vi "createTSR.vi"(0 "reference in":refnum<class "Project Panels.lvclass">=refnum, 5 "data":string[][](array[string]), 11 "error in (no error)":errorcluster) -> (4 "reference out":refnum<class "Project Panels.lvclass">, 8 "saved?":bool=TRUE, 15 "error out":errorcluster)   [LabVIEW 2015, in "Project Panels.lvclass"]
uses:
  Project Panels.lvclass
  tsrState.ctl
  SYS/File Controller_llb/File Controller.lvclass
  APP/excelFile_class/excelFile.lvclass
panel:
  out "PDF_path":path
  out "latest_TSR_path":string
  out "title":string="TSR"
  in  "End hour:":string(combo)="11:00"
  in  "Service Location:":bool
  in  "Start hour:":string(combo)="10:00" caption="start_hour"
  in  "PMC number:":string
  in  "Serial Number:":string
  in  "Device type:":T1(ring)
  in  "Service type:":string(combo)="Repair"
  in  "Discount (AUD):":i32
  in  "Shipping:":i32
  in  "Actions:":string
  in  "Contact:":string
  in  "Country:":string
  in  "Post Code:":string
  in  "City and State:":string
  in  "Department:":string
  in  "Issue description:":string
  in  "Address:":string
  in  "Company/Institution:":string
  in  "Parts:":string[][](table)=[["", ""]]
  in  "done":bool
  out "Status bar":string="Stop pressed"
  in  "Stop Button":bool
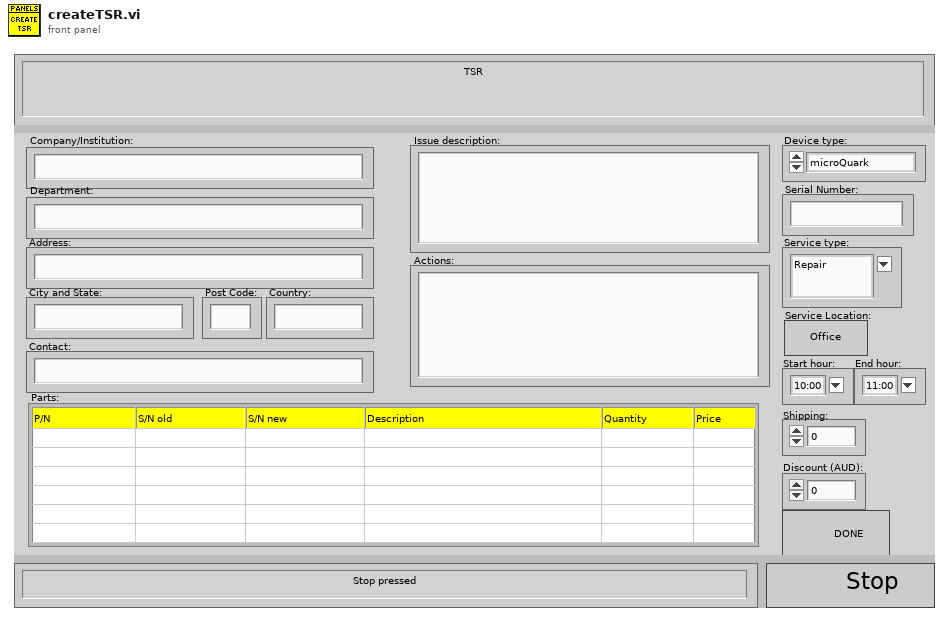
[diagram p1: front panel]
types:
  T1 = enum16{"microQuark", "Pony FX", "Spiropalm", "Spiropalm 6MWT", "PFT", "Body Box", "Fitmate PRO", "Fitmate WM", "Fitmate MED", "CPET", "RMR", "K4b2", "K5", "Bod Pod", "Pea Pod", "T12x", "C12x"}
  T2 = cluster{"Company/Institution:":string, "Address:":string, "Department:":string, "City:":string, "Post Code:":string, "Country:":string, "Contact:":string, "Ref:":string, "Issue description:":string, "Actions:":string, "TYPE:":string, "Shipping:":i32, "Discount:":i32, "dataIN":string[][], "Device type:":string, "Serial Number:":string, "PMC number:":string, "Labour Hours:":dbl, "Service Location:":bool, "start_hour":string, "end_hour":string}
  T3 = typedef "Project Panels.lvclass/tsrState.ctl" = enum16{"initiate", "waitEvent", "checkData", "checkFolders", "createTSR", "printTSR", "sendEmail", "stop", "close"}
  T4 = typedef "Project Panels.lvclass/ObjectAttributesRef.ctl" = refnum<data-value>
  T5 = typedef "Project Panels.lvclass/ObjectAttributes.ctl" = cluster{"MyAttribute":dbl, "device_controller_ref":refnum<class "Devices Controller.lvclass">, "file_controller_ref":refnum<class "File Controller.lvclass">, "item_controller_ref":refnum<class "Items Controller.lvclass">, "item_tables":cluster{"checkIN":string[][], "checkOUT":string[][], "storage":string[][]}, "quickbook_table":cluster{"notes":string[][]}, "notification_controller_ref":refnum<class "Notification Controller.lvclass">, "partstracking_controller_ref":refnum<class "PartsTracking Controller.lvclass">, "product_tables":cluster{"k4b2":string[][], "fitmate":string[][], "RMR":string[][], "CPET":string[][], "BP":string[][], "PP":string[][], "k5":string[][], "bb-pft":string[][]}, "rowsColour":u32[], "low_resolution?":bool, "run_python?":bool}
  T6 = cluster{"number":string, "TSR_path":path, "service_path":path, "email_to":string}
  T7 = enum16{"Left Button", "Center Button", "Right Button", "Window Close"}
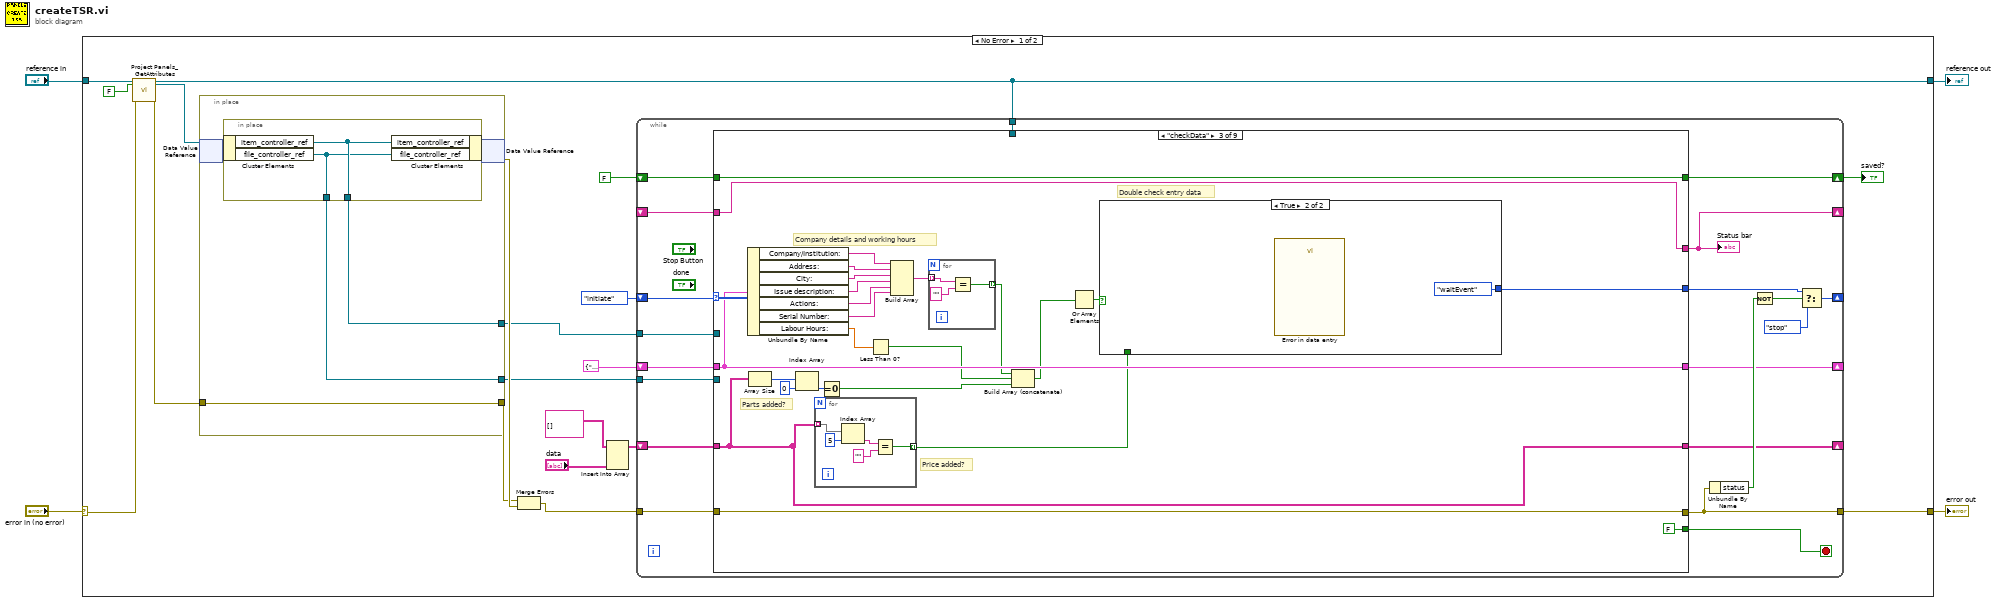
[diagram p0: block diagram]
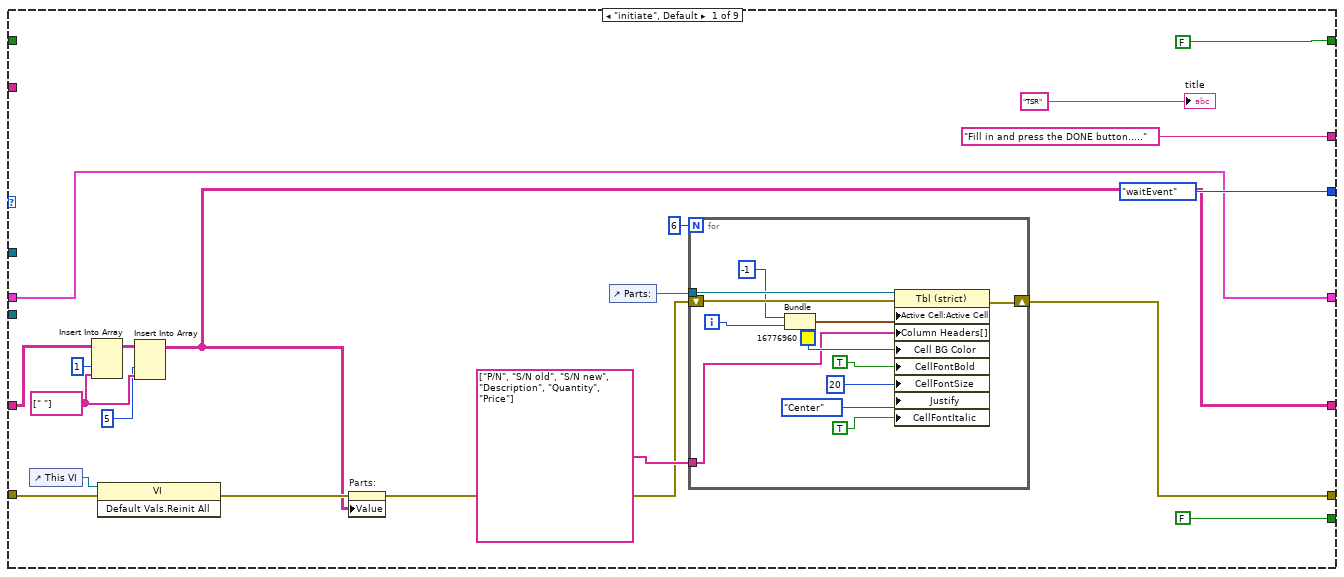
[diagram p2: hidden frame]
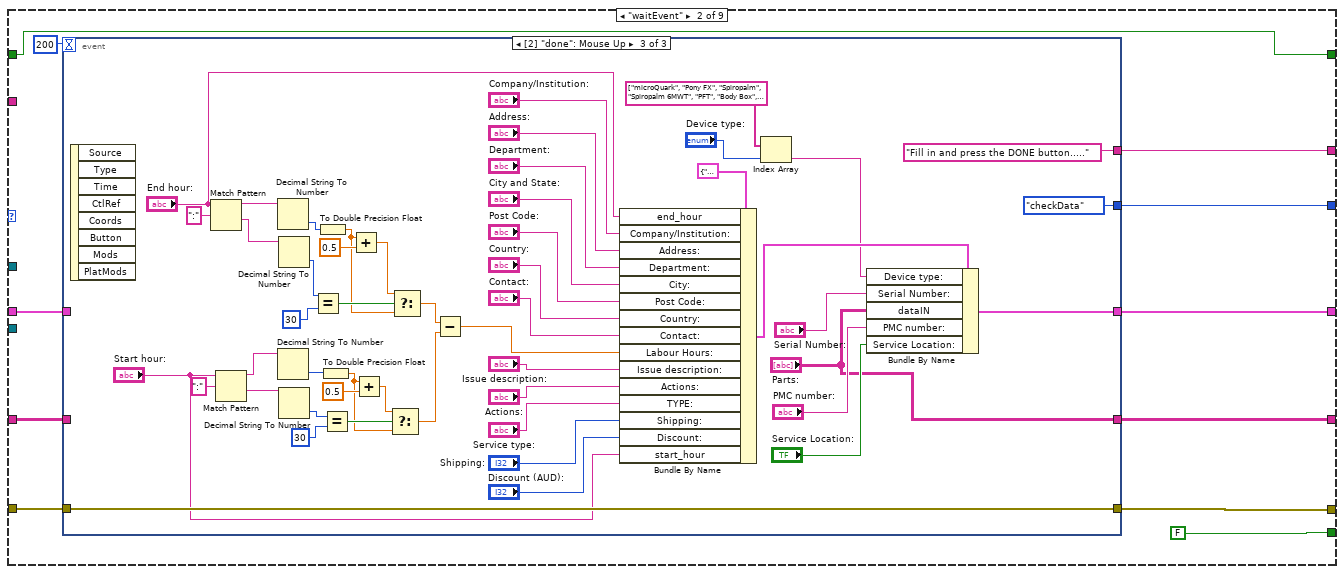
[diagram p3: hidden frame]
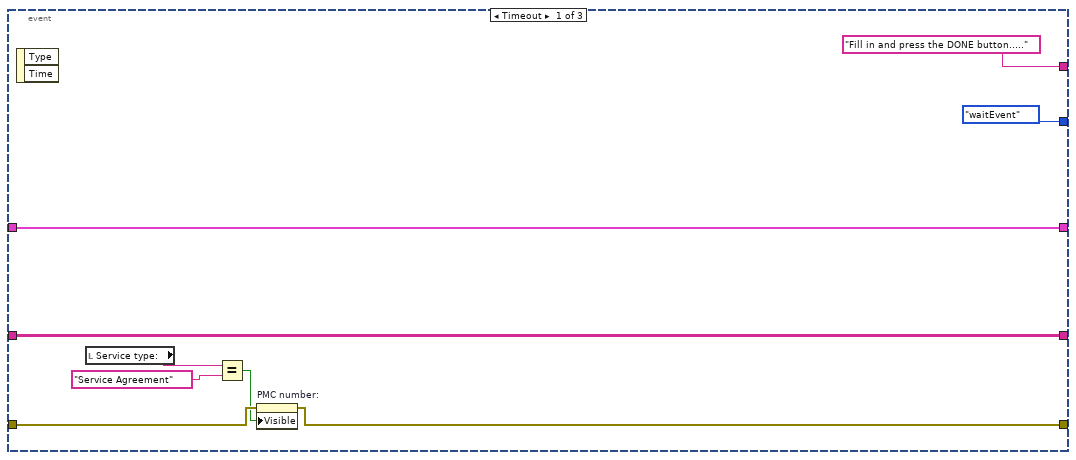
[diagram p4: hidden frame]
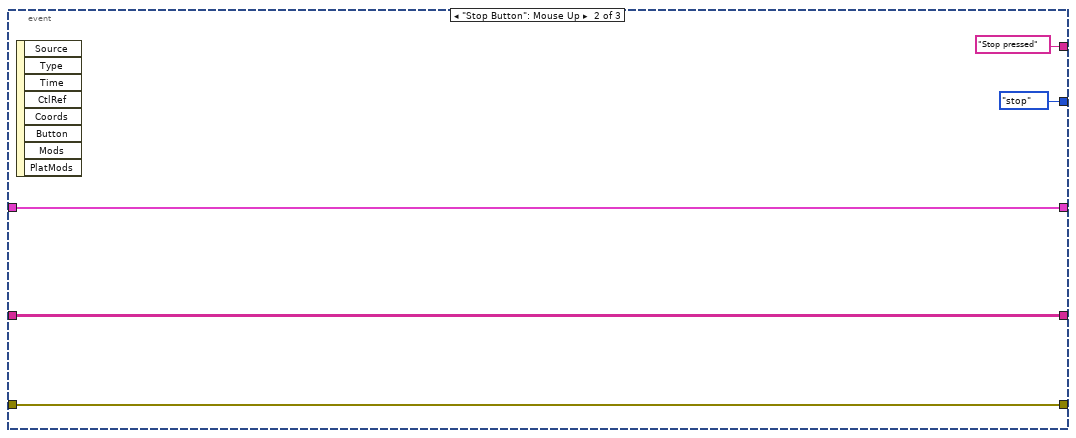
[diagram p5: hidden frame]
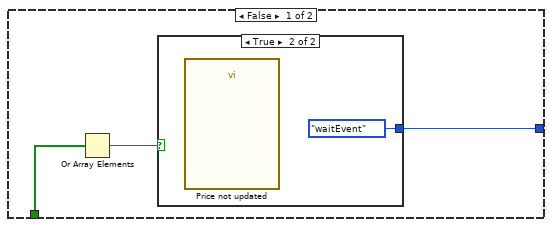
[diagram p6: hidden frame]
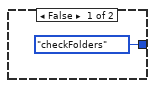
[diagram p7: hidden frame]
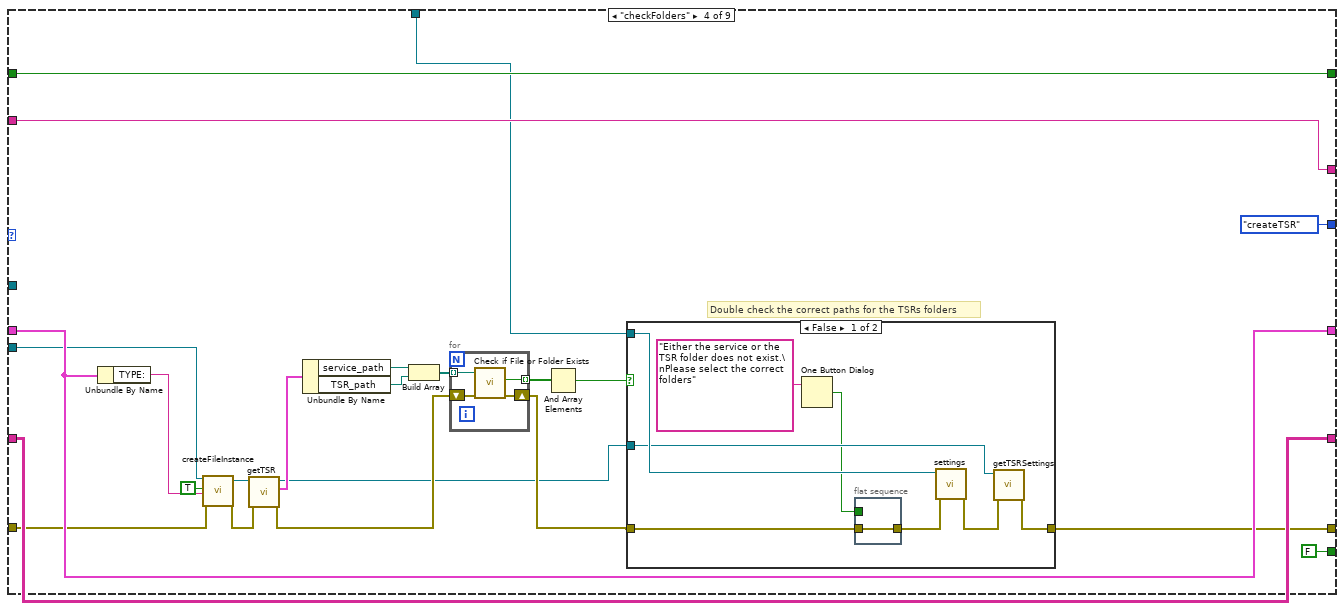
[diagram p8: hidden frame]
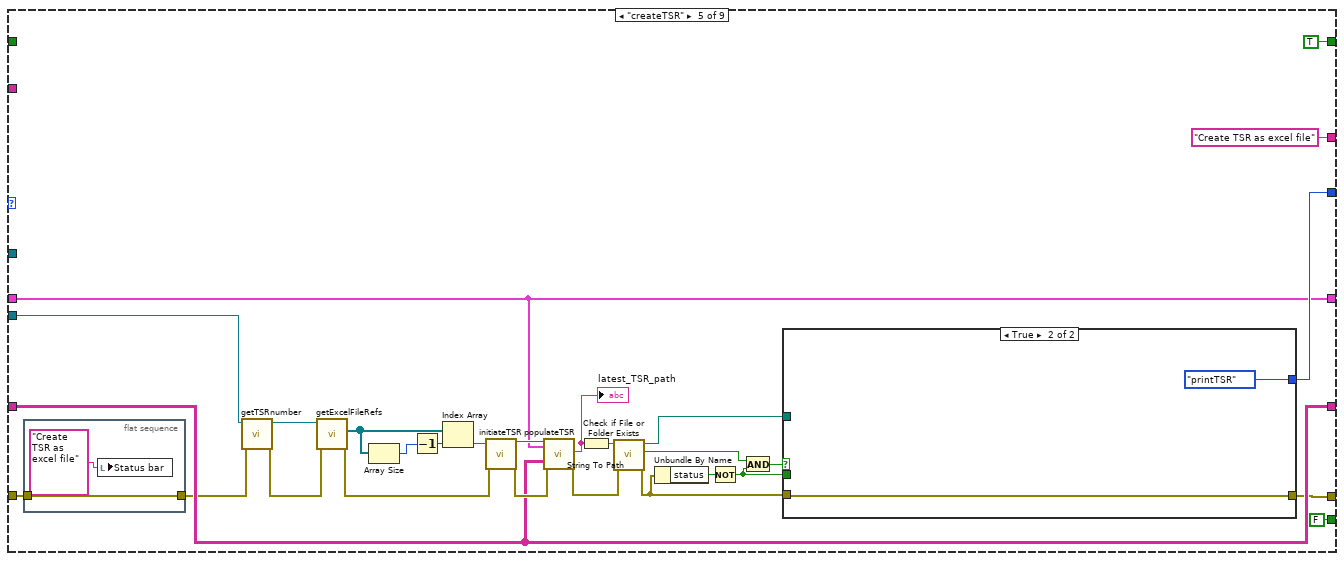
[diagram p10: hidden frame]
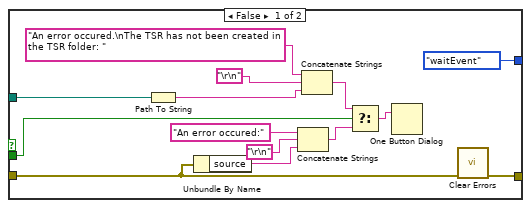
[diagram p11: hidden frame]
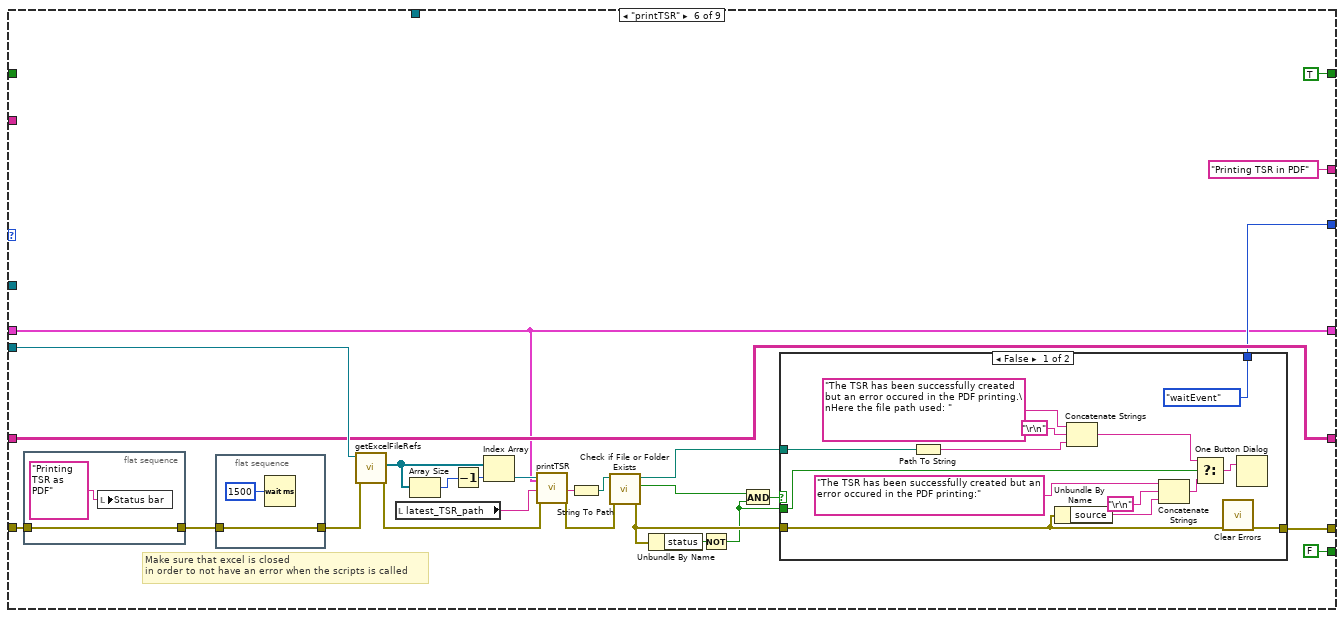
[diagram p12: hidden frame]
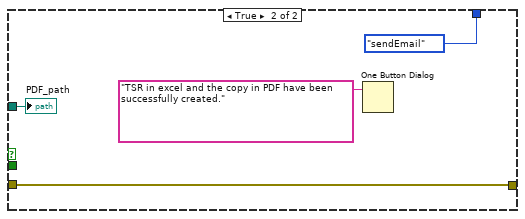
[diagram p13: hidden frame]
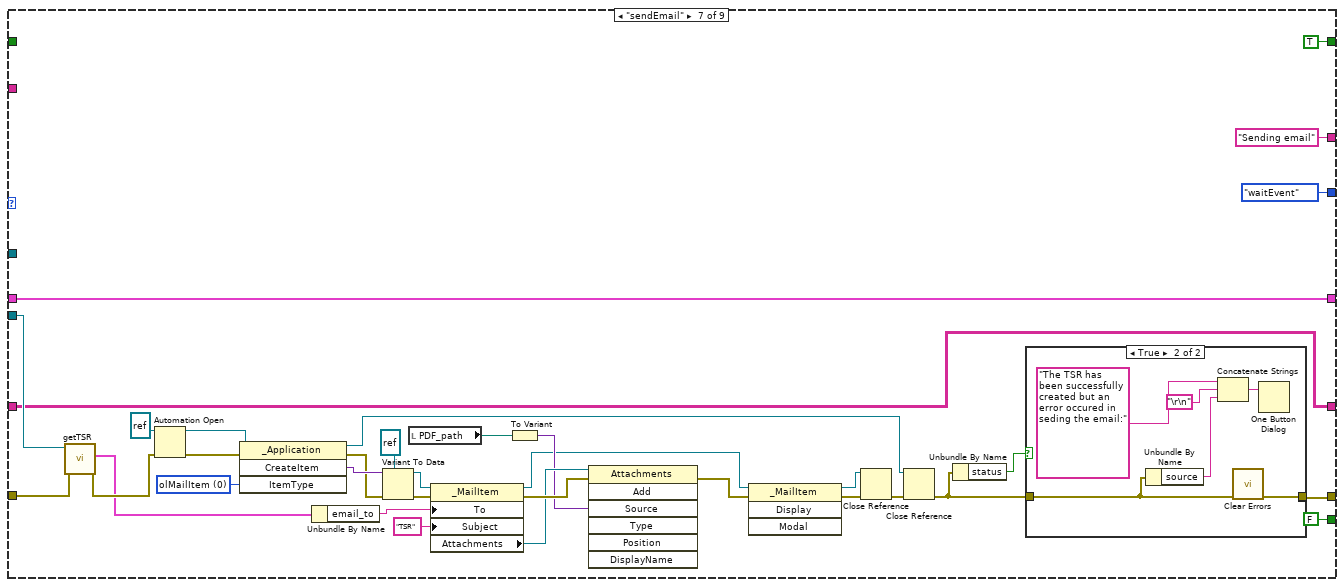
[diagram p14: hidden frame]
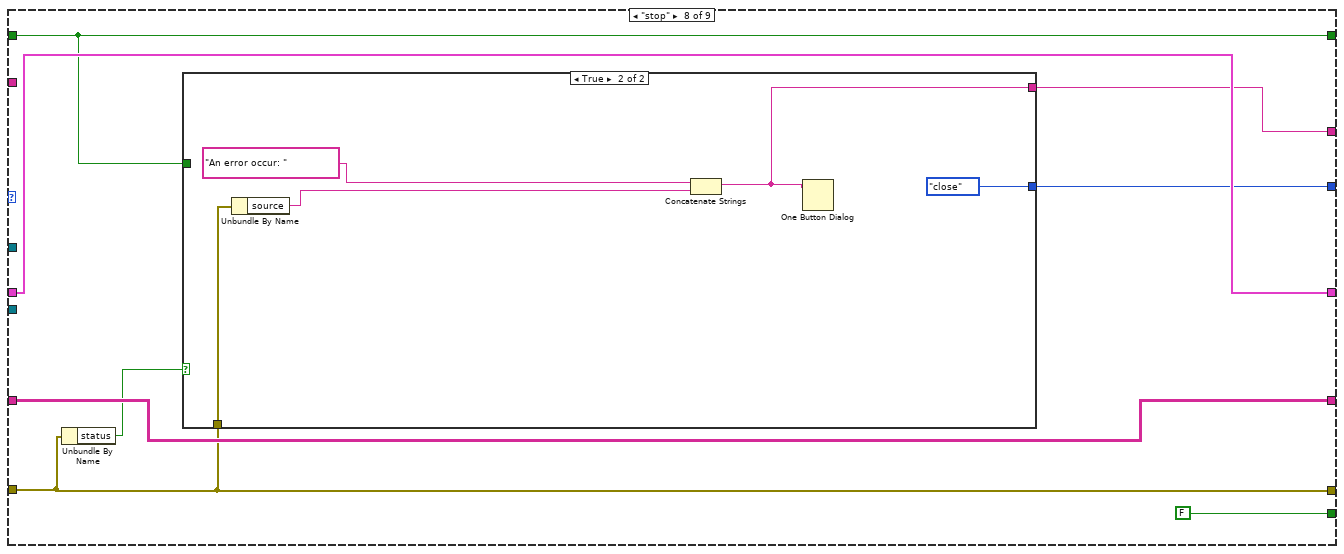
[diagram p16: hidden frame]
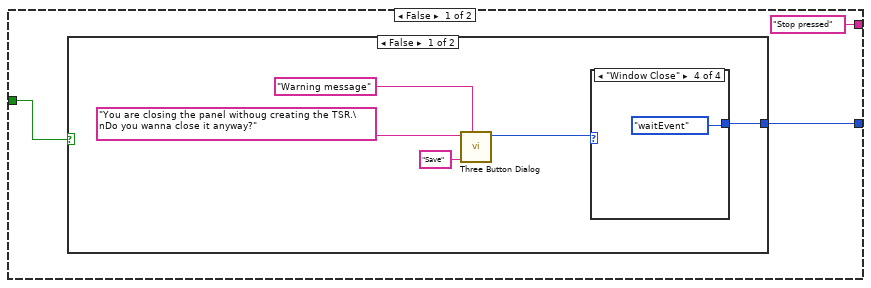
[diagram p17: hidden frame]
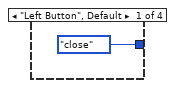
[diagram p18: hidden frame]
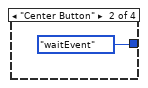
[diagram p19: hidden frame]
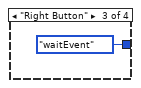
[diagram p20: hidden frame]
diagram:
  n1 = case shown="No Error" "error in (no error)" {
    selector: "error in (no error)" -> [w19 w402]
    tunnel: [w16 w402] -> w3
    tunnel: [w11 w401] -> w1
    tunnel: "reference in" -> [w21 w401]
    frame No Error {
      n2 = call "Project Panels_GetAttributes.vi"("reference in"=w21, "return data? (T)"=FALSE, "error in (no error)"=w19) -> ("reference out"=w11:refnum<class "Project Panels.lvclass">, "attributes ref"=w17:T4, "error out"=w18:errorcluster)  [unwired: 13 in, 1 out]
      n3 = in-place {
        in-place-border: w18 -> [w396]
        in-place-border: [w396] -> w22
        in-place-border: [w395] -> w14
        in-place-border: [w394] -> w10
        n4 = in-place-dvr #1(w17) -> (w397:T5)  [unwired: 1 out]
        n5 = in-place {
          in-place-border: [w400] -> w395
          in-place-border: [w399] -> w394
          n6 = in-place-cluster #2(w397) -> ("item_controller_ref"=w400:refnum<class "Items Controller.lvclass">, "file_controller_ref"=w399:refnum<class "File Controller.lvclass">)
          n7 = in-place-cluster #2("item_controller_ref"=w400, "file_controller_ref"=w399) -> (w398:T5)
        }
        n8 = in-place-dvr #1(w398) -> (w23:errorcluster)  [unwired: 1 out]
      }
      n9 = Merge Errors(w22, w23) -> (w9:errorcluster)
      n10 = Insert Into Array(array=string[][] [], new element="data") -> (w6:string[][])  [unwired: 2 in]
      n11 = while {
        tunnel: w9 -> [w35]
        tunnel: [w34] -> w16
        shift-right: [w43] -> _
        shift-left: tsrState."initiate" ("state") -> [w39]
        tunnel: w14 -> [w37]
        shift-right: [w33] -> _
        shift-left: w6 -> [w36]
        shift-right: [w31] -> w12
        shift-left: FALSE -> [w38]
        tunnel: w11 -> [w24]
        shift-right: [w29] -> _
        shift-left: T2 {"Company/Institution:"="", "Address:"="", "Department:"="", "City:"="", "Post Code:"="", "Country:"="", "Contact:"="", "Ref:"="", "Issue description:"="", "Actions:"="", "TYPE:"="Repair", "Shipping:"=0, "Discount:"=0, "dataIN"=[], "Device type:"="microQuark", "Serial Number:"="", "PMC number:"="", "Labour Hours:"=0.0, "Service Location:"=FALSE, "start_hour"="", "end_hour"=""} ("Cluster") -> [w28]
        shift-right: [w27] -> _
        shift-left: _ -> [w26]
        tunnel: w10 -> [w25]
        stop <- w30 stop-if-true
        n12 = case shown="\"checkData\"" w39 {
          tunnel: w38 -> [_ w79 w174 w211 _ _ _ w365 w391]
          tunnel: w37 -> [_ _ _ _ _ _ _ _ _]
          tunnel: w36 -> [w51 w81 w153 w209 w244 w276 w322 w367 w392]
          tunnel: w35 -> [w58 w83 w163 w204 w242 w294 w339 w364 w393]
          tunnel: [w57 w82 w163 w198 w241 w277 w323 w364 w393] -> w34
          tunnel: [w44 w80 w153 w209 w244 w276 w322 w367 w392] -> w33
          tunnel: [tsrState."waitEvent" ("state") w78 w165 tsrState."createTSR" ("state") w237 w274 tsrState."waitEvent" ("state") w362 tsrState."initiate" ("state")] -> w32
          tunnel: [FALSE w79 w174 w211 TRUE TRUE TRUE w365 w391] -> w31
          tunnel: ["Fill in and press the DONE button....." ("Status bar") w84 w151 w210 "Create TSR as excel file" ("Status bar") "Printing TSR in PDF" ("Status bar") "Sending email" ("Status bar") w361 w387] -> w27
          tunnel: [FALSE FALSE FALSE FALSE FALSE FALSE FALSE FALSE TRUE] -> w30
          tunnel: [w52 w77 w164 w207 w226 w272 w349 w366 w388] -> w29
          tunnel: w28 -> [w52 w76 w164 w207 w226 w272 w349 w366 w388]
          tunnel: w26 -> [_ _ w151 w210 _ _ _ _ w387]
          tunnel: w25 -> [_ _ _ w201 w235 w289 w340 _ _]
          tunnel: w24 -> [_ _ _ w191 _ _ _ _ _]
          frame "initiate", Default {
            w48 = string[] [" "] ("new element/subarray")
            n13 = control-ref of="This VI"() -> (w60:refnum<vi>)
            n14 = Insert Into Array(array=w51, index (col)=1 ("disabled index (col)"), new element=w48) -> (w49:string[][])  [unwired: 1 in]
            n15 = invoke class="VI" method="Default Vals.Reinit All"(reference=w60, error in=w58) -> (error out=w46:errorcluster)  [unwired: 1 in, 2 out]
            n16 = Insert Into Array(array=w49, index (col)=5 ("disabled index (col)"), new element=w48) -> (w44:string[][])  [unwired: 1 in]
            n17 = property on="Parts:" class="Tbl (strict)"(error in=w46, "Value"=w44) -> (error out=w45:errorcluster)  [unwired: 1 in, 1 out]
            n18 = control-ref of="Parts:"() -> (w63:refnum<vi>)
            n19 = for {
              N: 6 -> [_]
              tunnel: w63 -> [w73]
              shift-right: [w74] -> w57
              shift-left: w45 -> [w75]
              tunnel: string[] ["P/N", "S/N old", "S/N new", "Description", "Quantity", "Price"] ("Column Header Strings[]") -> [w64]
              i -> [w71]
              n20 = Bundle("index"=-1, w71) -> (w72:cluster{"index":i32, i32})  [unwired: 1 in]
              n21 = property on="Property Node" class="Tbl (strict)"(reference=w73, error in=w75, "Active Cell:Active Cell"=w72, "Column Headers[]"=w64, "Cell BG Color"=u32 16776960, "CellFontBold"=TRUE ("Active Cell:Cell Font:Bold"), "CellFontSize"=u32 20 ("Active Cell:Cell Font:Size"), "Justify"=enum16{"Left", "Center", "Right"}."Center" ("Active Cell:Cell Justification"), "CellFontItalic"=TRUE ("Active Cell:Cell Font:Italic")) -> (error out=w74:errorcluster)  [unwired: 1 out]
            }
            "title" <- "TSR" ("title")
          }
          frame "waitEvent" {
            n22 = event shown="[2] \"done\": Mouse Up" {
              selector: _ -> [_ _ _]
              dyn-events: _ -> [_ _ _]
              timeout: 200 -> [_ _ _]
              tunnel: [tsrState."waitEvent" ("state") tsrState."stop" ("state") tsrState."checkData" ("state")] -> w78
              tunnel: ["Fill in and press the DONE button....." ("Status bar") "Stop pressed" ("Status bar") "Fill in and press the DONE button....." ("Status bar")] -> w84
              tunnel: w83 -> [w89 w97 w149]
              tunnel: [w88 w97 w149] -> w82
              tunnel: w81 -> [w93 w98 _]
              tunnel: [w93 w98 "Parts:"] -> w80
              tunnel: [w92 w96 w138] -> w77
              tunnel: w76 -> [w92 w96 _]
              event Timeout {
                n23 = event-data() -> ()  [unwired: 1 in, 2 out]
                n24 = local read "Service type:"() -> (w90:string)
                n25 = Equal?(x=w90, y="Service Agreement" ("TYPE:")) -> (x = y?=w87:bool)
                n26 = property on="PMC number:" class="Str"(error in=w89, "Visible"=w87) -> (error out=w88:errorcluster)  [unwired: 1 in, 1 out]
              }
              event "Stop Button": Mouse Up {
                n27 = event-data() -> ()  [unwired: 1 in, 8 out]
              }
              event "done": Mouse Up {
                n28 = event-data() -> ()  [unwired: 1 in, 8 out]
                n29 = Match Pattern(string="End hour:", regular expression=":") -> (before substring=w122:string, after substring=w105:string)  [unwired: 1 in, 2 out]
                n30 = Match Pattern(string="Start hour:", regular expression=":") -> (before substring=w124:string, after substring=w123:string)  [unwired: 1 in, 2 out]
                n31 = Decimal String To Number(string=w122) -> (number=w115:i32)  [unwired: 2 in, 1 out]
                n32 = Decimal String To Number(string=w124) -> (number=w108:i32)  [unwired: 2 in, 1 out]
                n33 = Decimal String To Number(string=w105) -> (number=w118:i32)  [unwired: 2 in, 1 out]
                n34 = Decimal String To Number(string=w123) -> (number=w121:i32)  [unwired: 2 in, 1 out]
                n35 = Equal?(x=w118, y=30) -> (x = y?=w116:bool)
                n36 = To Double Precision Float(number=w115) -> (double precision float=w112:dbl)
                n37 = To Double Precision Float(number=w108) -> (double precision float=w107:dbl)
                n38 = Equal?(x=w121, y=30) -> (x = y?=w119:bool)
                n39 = Add(x=w112, y=0.5) -> (x+y=w113:dbl)
                n40 = Add(x=w107, y=0.5) -> (x+y=w109:dbl)
                n41 = Select(t=w109, s=w119, f=w107) -> (s? t:f=w106:dbl)
                n42 = Select(t=w113, s=w116, f=w112) -> (s? t:f=w111:dbl)
                n43 = Subtract(x=w111, y=w106) -> (x-y=w104:dbl)
                n44 = Bundle By Name(cluster=T2 {"Company/Institution:"="", "Address:"="", "Department:"="", "City:"="", "Post Code:"="", "Country:"="", "Contact:"="", "Ref:"="", "Issue description:"="", "Actions:"="", "TYPE:"="Repair", "Shipping:"=0, "Discount:"=0, "dataIN"=[], "Device type:"="microQuark", "Serial Number:"="", "PMC number:"="", "Labour Hours:"=0.0, "Service Location:"=FALSE, "start_hour"="", "end_hour"=""} ("Cluster"), "end_hour"="End hour:", "Company/Institution:"="Company/Institution:", "Address:"="Address:", "Department:"="Department:", "City:"="City and State:", "Post Code:"="Post Code:", "Country:"="Country:", "Contact:"="Contact:", "Labour Hours:"=w104, "Issue description:"="Issue description:", "Actions:"="Actions:", "TYPE:"="Service type:", "Shipping:"="Shipping:", "Discount:"="Discount (AUD):", "start_hour"="Start hour:") -> (w140:T2)
                n45 = Index Array(array=string[] ["microQuark", "Pony FX", "Spiropalm", "Spiropalm 6MWT", "PFT", "Body Box", "Fitmate PRO", "Fitmate WM", "Fitmate MED", "CPET", "RMR", "K4b2", "K5", "Bod Pod", "Pea Pod", "T12x", "C12x"], index="Device type:") -> (element=w127:string)
                n46 = Bundle By Name(cluster=w140, "Device type:"=w127, "Serial Number:"="Serial Number:", "dataIN"="Parts:", "PMC number:"="PMC number:", "Service Location:"="Service Location:") -> (w138:T2)
              }
            }
          }
          frame "checkData" {
            # "Price added?"
            # "Parts added?"
            # "Company details and working hours"
            # "Double check entry data"
            n47 = Unbundle By Name(w164) -> ("Company/Institution:"=w172:string, "Address:"=w171:string, "City:"=w170:string, "Issue description:"=w169:string, "Actions:"=w168:string, "Serial Number:"=w167:string, "Labour Hours:"=w162:dbl)
            n48 = Array Size(array=w153) -> (size(s)=w161:i32[])
            n49 = Index Array(array=w161, index=0) -> (element=w159:i32)
            n50 = for {
              tunnel: w153 -> [w179] mode=indexing
              tunnel: [w175] -> w152 mode=indexing
              n51 = Index Array(array=w179, index=5) -> (element=w176:string)
              n52 = Equal?(x=w176, y="") -> (x = y?=w175:bool)
            }
            n53 = Equal To 0?(x=w159) -> (x = 0?=w156:bool)
            n54 = Less Than 0?(x=w162) -> (x < 0?=w157:bool)
            n55 = Build Array(w172, w171, w170, w169, w168, w167) -> (w166:string[])
            n56 = for {
              tunnel: w166 -> [w188] mode=indexing
              tunnel: [w186] -> w158 mode=indexing
              n57 = Equal?(x=w188, y="") -> (x = y?=w186:bool)
            }
            n58 = Build Array (concatenate)(w158, w157, w156) -> (w154:bool[])
            n59 = Or Array Elements(Boolean array=w154) -> (logical OR=w155:bool)
            n60 = case shown="True" w155 {
              tunnel: [w180 tsrState."waitEvent" ("state")] -> w165
              tunnel: w152 -> [w182 _]
              frame False {
                n61 = Or Array Elements(Boolean array=w182) -> (logical OR=w181:bool)
                n62 = case shown="True" w181 {
                  tunnel: [tsrState."checkFolders" ("state") tsrState."waitEvent" ("state")] -> w180
                  frame False {
                  }
                  frame True {
                    n63 = call "Price not updated"() -> ()  [unwired: 10 in, 2 out]
                  }
                }
              }
              frame True {
                n64 = call "Error in data entry"() -> ()  [unwired: 10 in, 2 out]
              }
            }
          }
          frame "checkFolders" {
            # "Double check the correct paths for the TSRs folders"
            n65 = Unbundle By Name(w207) -> ("TYPE:"=w206:string)
            n66 = call "createFileInstance.vi"("reference in"=w201, "TSR?"=TRUE, "TYPE:"=w206, "error in (no error)"=w204) -> ("reference out"=w202:refnum<class "File Controller.lvclass">, "error out"=w203:errorcluster)  [unwired: 14 in]
            n67 = call "getTSR.vi"("error in (no error)"=w203, "reference in"=w202) -> ("error out"=w193:errorcluster, "TSR"=w197:T6, "reference out"=w190:refnum<class "File Controller.lvclass">)  [unwired: 7 in]
            n68 = Unbundle By Name(w197) -> ("service_path"=w200:path, "TSR_path"=w199:path)
            n69 = Build Array(w200, w199) -> (w196:path[])
            n70 = for {
              tunnel: w196 -> [w215] mode=indexing
              tunnel: [w214] -> w195 mode=indexing
              shift-right: [w212] -> w192
              shift-left: w193 -> [w213]
              n71 = call <vilib>:"Check if File or Folder Exists.vi"("error in (no error)"=w213, "path"=w215) -> ("error out"=w212:errorcluster, "file or folder exists?"=w214:bool)  [unwired: 7 in, 1 out]
            }
            n72 = And Array Elements(Boolean array=w195) -> (logical AND=w194:bool)
            n73 = case shown="False" w194 {
              tunnel: w192 -> [w218 w225]
              tunnel: [w220 w225] -> w198
              tunnel: w191 -> [w222 _]
              tunnel: w190 -> [w219 _]
              frame False {
                n74 = One Button Dialog(message="Either the service or the TSR folder does not exist.\nPlease select the correct folders") -> (true=w216:bool)  [unwired: 1 in]
                n75 = flat-sequence {
                  tunnel: w218 -> [w224]
                  tunnel: [w224] -> w217
                  tunnel: w216 -> [_]
                  frame #0 {
                  }
                }
                n76 = call "settings.vi"("error in (no error)"=w217, "reference in"=w222) -> ("error out"=w221:errorcluster)  [unwired: 8 in, 1 out]
                n77 = call "getTSRSettings.vi"("error in (no error)"=w221, "reference in"=w219) -> ("error out"=w220:errorcluster)  [unwired: 8 in, 1 out]
              }
              frame True {
              }
            }
          }
          frame "createTSR" {
            n78 = flat-sequence {
              tunnel: w242 -> [w271]
              tunnel: [w271] -> w236
              frame #0 {
                n79 = local write "Status bar"("Create TSR as excel file" ("Status bar")) -> ()
              }
            }
            n80 = call "getTSRnumber.vi"("error in (no error)"=w236, "reference in"=w235) -> ("error out"=w246:errorcluster, "reference out"=w245:refnum<class "File Controller.lvclass">)  [unwired: 8 in]
            n81 = call "getExcelFileRefs.vi"("error in (no error)"=w246, "reference in"=w245) -> ("error out"=w233:errorcluster, "excelFile_refs"=w250:refnum<class "excelFile.lvclass">[])  [unwired: 7 in, 1 out]
            n82 = Array Size(array=w250) -> (size(s)=w249:i32)
            n83 = Decrement(x=w249) -> (x-1=w243:i32)
            n84 = Index Array(array=w250, index=w243) -> (element=w234:refnum<class "excelFile.lvclass">)
            n85 = call "initiateTSR.vi"("reference in"=w234, "error in (no error)"=w233) -> ("reference out"=w248:refnum<class "excelFile.lvclass">, "error out"=w247:errorcluster)  [unwired: 16 in]
            n86 = call "populateTSR.vi"("reference in"=w248, "TSR_details"=w226, "data"=w244, "error in (no error)"=w247) -> ("latest_TSR_path"=w240:string, "error out"=w238:errorcluster)  [unwired: 13 in, 1 out]
            "latest_TSR_path" <- w240
            n87 = String To Path(string=w240) -> (path=w239:path)
            n88 = call <vilib>:"Check if File or Folder Exists.vi"("error in (no error)"=w238, "path"=w239) -> ("error out"=w232:errorcluster, "file or folder exists?"=w231:bool, "dup path"=w228:path)  [unwired: 7 in]
            n89 = Unbundle By Name(w232) -> ("status"=w229:bool)
            n90 = Not(x=w229) -> (.not. x?=w227:bool)
            n91 = And(x=w231, y=w227) -> (x .and. y?=w230:bool)
            n92 = case shown="True" w230 {
              tunnel: [w254 w268] -> w241
              tunnel: w232 -> [w255 w268]
              tunnel: [tsrState."waitEvent" ("state") tsrState."printTSR" ("state")] -> w237
              tunnel: w227 -> [w266 _]
              tunnel: w228 -> [w264 _]
              frame False {
                n93 = Path To String(path=w264) -> (string=w262:string)
                n94 = Unbundle By Name(w255) -> ("source"=w258:string)
                n95 = Concatenate Strings("An error occured:", "\r\n", w258) -> (w260:string)
                n96 = Concatenate Strings("An error occured.\nThe TSR has not been created in the TSR folder: ", "\r\n", w262) -> (w263:string)
                n97 = Select(t=w263, s=w266, f=w260) -> (s? t:f=w256:string)
                n98 = One Button Dialog(message=w256) -> ()  [unwired: 1 in, 1 out]
                n99 = call <vilib>:"Clear Errors.vi"("error in (no error)"=w255) -> ("error out"=w254:errorcluster)  [unwired: 5 in, 1 out]
              }
              frame True {
              }
            }
          }
          frame "printTSR" {
            # "Make sure that excel is closed \nin order to not have an error when the scripts is called"
            n100 = flat-sequence {
              tunnel: w294 -> [w317]
              tunnel: [w317] -> w293
              frame #0 {
                n101 = local write "Status bar"("Printing TSR as PDF" ("Status bar")) -> ()
              }
            }
            n102 = flat-sequence {
              tunnel: w293 -> [w318]
              tunnel: [w318] -> w288
              frame #0 {
                n103 = Wait (ms)(milliseconds to wait=u32 1500) -> ()  [unwired: 1 out]
              }
            }
            n104 = call "getExcelFileRefs.vi"("error in (no error)"=w288, "reference in"=w289) -> ("error out"=w287:errorcluster, "excelFile_refs"=w292:refnum<class "excelFile.lvclass">[])  [unwired: 7 in, 1 out]
            n105 = local read "latest_TSR_path"() -> (w285:string)
            n106 = Array Size(array=w292) -> (size(s)=w291:i32)
            n107 = Decrement(x=w291) -> (x-1=w290:i32)
            n108 = Index Array(array=w292, index=w290) -> (element=w286:refnum<class "excelFile.lvclass">)
            n109 = call "printTSR.vi"("reference in"=w286, "TSR_details"=w272, "latest_TSR_path"=w285, "error in (no error)"=w287) -> ("PDF_file_path"=w281:string, "error out"=w284:errorcluster)  [unwired: 13 in, 1 out]
            n110 = String To Path(string=w281) -> (path=w280:path)
            n111 = call <vilib>:"Check if File or Folder Exists.vi"("error in (no error)"=w284, "path"=w280) -> ("error out"=w278:errorcluster, "file or folder exists?"=w282:bool, "dup path"=w279:path)  [unwired: 7 in]
            n112 = Unbundle By Name(w278) -> ("status"=w275:bool)
            n113 = Not(x=w275) -> (.not. x?=w273:bool)
            n114 = And(x=w282, y=w273) -> (x .and. y?=w283:bool)
            n115 = case shown="False" w283 {
              tunnel: [w308 w315] -> w277
              tunnel: w278 -> [w309 w315]
              tunnel: w273 -> [w311 _]
              tunnel: w279 -> [w310 w312]
              tunnel: [tsrState."waitEvent" ("state") tsrState."sendEmail" ("state")] -> w274
              frame False {
                n116 = Path To String(path=w310) -> (string=w304:string)
                n117 = Unbundle By Name(w309) -> ("source"=w300:string)
                n118 = Concatenate Strings("The TSR has been successfully created but an error occured in the PDF printing.\nHere the file path used: ", "\r\n", w304) -> (w305:string)
                n119 = Concatenate Strings("The TSR has been successfully created but an error occured in the PDF printing:", "\r\n", w300) -> (w302:string)
                n120 = Select(t=w305, s=w311, f=w302) -> (s? t:f=w298:string)
                n121 = call <vilib>:"Clear Errors.vi"("error in (no error)"=w309) -> ("error out"=w308:errorcluster)  [unwired: 5 in, 1 out]
                n122 = One Button Dialog(message=w298) -> ()  [unwired: 1 in, 1 out]
              }
              frame True {
                n123 = One Button Dialog(message="TSR in excel and the copy in PDF have been successfully created.") -> ()  [unwired: 1 in, 1 out]
                "PDF_path" <- w312
              }
            }
          }
          frame "sendEmail" {
            w345 = 0 items=["olMailItem"=0, "olAppointmentItem"=1, "olContactItem"=2, "olTaskItem"=3, "olJournalItem"=4, "olNoteItem"=5, "olPostItem"=6, "olDistributionListItem"=7, "olMobileItemSMS"=11, "olMobileItemMMS"=12] ("ItemType")
            n124 = call "getTSR.vi"("error in (no error)"=w339, "reference in"=w340) -> ("error out"=w338:errorcluster, "TSR"=w337:T6)  [unwired: 7 in, 1 out]
            n125 = Automation Open(error in (no error)=w338, Automation Refnum=refnum<k7> refnum ("Outlook._Application")) -> (Automation Refnum=w348:refnum<k7>, error out=w347:errorcluster)  [unwired: 2 in]
            n126 = invoke class="_Application" method="CreateItem"(reference=w348, error in=w347, "ItemType"=w345) -> (reference out=w324:refnum<k7>, error out=w342:errorcluster, "CreateItem"=w344:variant)  [unwired: 1 in, 1 out]
            n127 = Unbundle By Name(w337) -> ("email_to"=w336:string)
            n128 = Variant To Data(error in=w342, type=refnum<k7> refnum ("Outlook._MailItem"), Variant=w344) -> (data=w330:refnum<k7>, error out=w341:errorcluster)
            n129 = local read "PDF_path"() -> (w332:path)
            n130 = property class="_MailItem"(reference=w330, error in=w341, "To"=w336, "Subject"="TSR") -> (reference out=w325:refnum<k7>, error out=w334:errorcluster, "Attachments"=w333:refnum<k7>)
            n131 = To Variant(anything=w332) -> (Variant=w331:variant)
            n132 = invoke class="Attachments" method="Add"(reference=w333, error in=w334, "Source"=w331) -> (error out=w326:errorcluster)  [unwired: 4 in, 6 out]
            n133 = invoke class="_MailItem" method="Display"(reference=w325, error in=w326) -> (reference out=w328:refnum<k7>, error out=w327:errorcluster)  [unwired: 2 in, 2 out]
            n134 = Close Reference(reference=w328, error in (no error)=w327) -> (error out=w329:errorcluster)
            n135 = Close Reference(reference=w324, error in (no error)=w329) -> (error out=w321:errorcluster)
            n136 = Unbundle By Name(w321) -> ("status"=w320:bool)
            n137 = case shown="True" w320 {
              tunnel: w321 -> [w354 w356]
              tunnel: [w354 w355] -> w323
              tunnel: w321 -> [_ _]
              frame False {
              }
              frame True {
                n138 = Unbundle By Name(w356) -> ("source"=w360:string)
                n139 = Concatenate Strings("The TSR has been successfully created but an error occured in seding the email:", "\r\n", w360) -> (w357:string)
                n140 = call <vilib>:"Clear Errors.vi"("error in (no error)"=w356) -> ("error out"=w355:errorcluster)  [unwired: 5 in, 1 out]
                n141 = One Button Dialog(message=w357) -> ()  [unwired: 1 in, 1 out]
              }
            }
          }
          frame "stop" {
            n142 = Unbundle By Name(w364) -> ("status"=w363:bool)
            n143 = case shown="True" w363 {
              tunnel: w364 -> [_ w384]
              tunnel: ["Stop pressed" w383] -> w361
              tunnel: [w370 tsrState."close" ("state")] -> w362
              tunnel: w365 -> [w369 _]
              frame False {
                n144 = case shown="False" w369 {
                  tunnel: [w372 tsrState."close" ("state")] -> w370
                  frame False {
                    n145 = call <vilib>:"Three Button Dialog.vi"("Window Title (\"\")"="Warning message" ("Window Title (\"\")"), "Right Button Text (\"Cancel\")"="Save" ("Right Button Text (\"Cancel\")"), "message"="You are closing the panel withoug creating the TSR.\nDo you wanna close it anyway?") -> ("Which Button?"=w373:T7)  [unwired: 8 in]
                    n146 = case shown="\"Window Close\"" w373 {
                      tunnel: [tsrState."close" ("state") tsrState."waitEvent" ("state") tsrState."waitEvent" ("state") tsrState."waitEvent" ("state")] -> w372
                      frame "Left Button", Default {
                      }
                      frame "Center Button" {
                      }
                      frame "Right Button" {
                      }
                      frame "Window Close" {
                      }
                    }
                  }
                  frame True {
                  }
                }
              }
              frame True {
                n147 = Unbundle By Name(w384) -> ("source"=w385:string)
                n148 = Concatenate Strings("An error occur: " ("message"), w385) -> (w383:string)
                n149 = One Button Dialog(message=w383) -> ()  [unwired: 1 in, 1 out]
              }
            }
          }
          frame "close" {
          }
        }
        "Status bar" <- w27
        n150 = Unbundle By Name(w34) -> ("status"=w42:bool)
        n151 = Not(x=w42) -> (.not. x?=w41:bool)
        n152 = Select(t=w32, s=w41, f=tsrState."stop" ("state")) -> (s? t:f=w43:T3)
      }
      "saved?" <- w12
    }
    frame Error {
    }
  }
  "error out" <- w3
  "reference out" <- w1
